vi "lvEtherbone.get shared library version.vi"(5 "error in (no error)":errorcluster) -> (15 "lvebVersion":string, 16 "ebVersion":string, 19 "error out":errorcluster)   [LabVIEW 2009, in "lvEtherbone.lvlib"]
doc: "//-----------------------------------------------------------------------------------\n// author : Dietrich Beck, GSI-Darmstadt\n// purpose : obtains version information about Etherbone shared library software.\n// The caller must preallocate sufficient memory.\n// returns : void\n//-----------------------------------------------------------------------------------\nETHERBONE_API void lveb_get_version( char *lvebVersion, //version of lvEtherbone library\n char *ebVersion //version of Etherbone API\n );"
uses:
  lvEtherbone.lvlib
  bin/lvEtherbone.dll
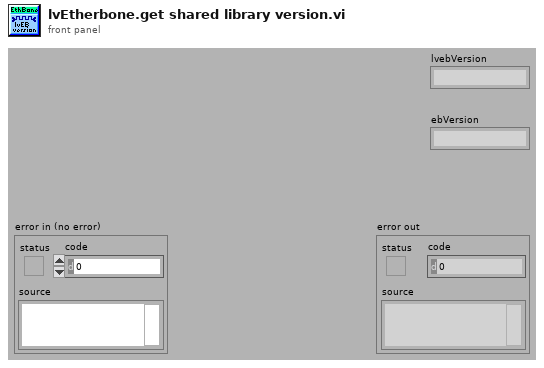
[diagram p1: front panel]
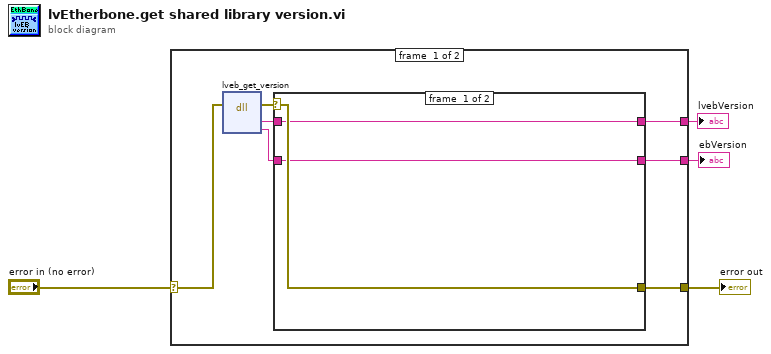
[diagram p0: block diagram]
diagram:
  n1 = case shown="No Error" "error in (no error)" {
    selector: "error in (no error)" -> [w11 w16]
    tunnel: [w9 w16] -> w3
    tunnel: [w7 _] -> w2
    tunnel: [w5 _] -> w1
    frame #0 {
      n2 = dll-call lib="F:/beck/Project/BEL/SCC/etherbone-core/api/lvEtherbone/bin/lvEtherbone.*" fn="lveb_get_version"(error in=w11) -> (error out=w10:errorcluster, "lvebVersion"=w8:string, "ebVersion"=w6:string)  [unwired: 5 in, 1 out]
      n3 = case shown="No Error" w10 {
        selector: w10 -> [w14 w15]
        tunnel: [w14 w15] -> w9
        tunnel: w8 -> [w13 _]
        tunnel: [w13 _] -> w7
        tunnel: w6 -> [w12 _]
        tunnel: [w12 _] -> w5
        frame #0 {
        }
        frame #1 {
        }
      }
    }
    frame #1 {
    }
  }
  "error out" <- w3
  "lvebVersion" <- w2
  "ebVersion" <- w1
